vi "DSCProgClient.vi"() -> ()   [LabVIEW 2011]
uses:
  <vilib>/variable/tagger/epics/API/internal/List Records (By Ref).vi
  <vilib>/variable/tagger/epics/API/internal/Undeploy EPICS Client (By Ref).vi
  <vilib>/variable/tagger/epics/API/NI_EPICS_Client.lvlib
  <vilib>/lvdsc/NI_DSC.lvlib
panel:
  in  "network settings":T1={"use binding? (F)"=TRUE, "URL"="\\\\ndw1032\\vlinac\\css\\css:cos\\VAL", "access type"=enum."Read/write", "buffer size"=50, "use buffering? (F)"=FALSE, "single writer? (F)"=FALSE}
  out "error out 2":errorcluster
  out "data out":dbl
  out "error out":errorcluster={"status"=TRUE, "code"=-1967362038, "source"="Search Variable Container in DSCProgClient.vi"}
  out "records":string[](array[string])=["css:cos"]
  in  "stop":bool
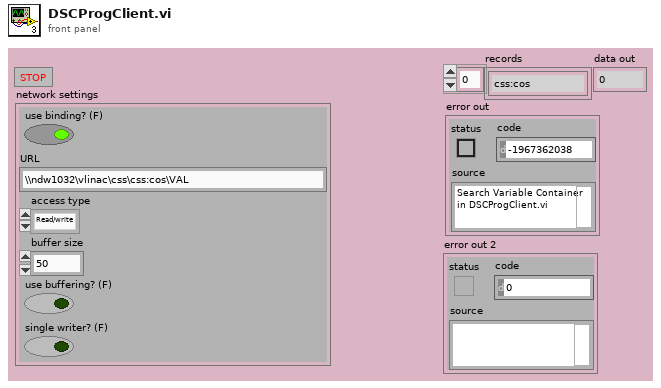
[diagram p1: front panel]
types:
  T1 = cluster{"use binding? (F)":bool, "URL":string, "access type":enum32{"Read only", "Write only", "Read/write"}, "buffer size":u32, "use buffering? (F)":bool, "single writer? (F)":bool}
  T2 = enum32{"u32BitField", "bool", "double", "string", "int8", "uint8", "int16", "uint16", "int32", "uint32", "int64", "uint64", "single", "double waveform", "int16 waveform", "array of boolean", "array of int8", "array of uint8", "array of int16", "array of uint16", "array of int32", "array of uint32", "array of int64", "array of uint64", "array of single", "array of double", "array of double waveform", "array of int16 waveform", "array of string", "variant", "timestamp", "fixed point", "custom"}
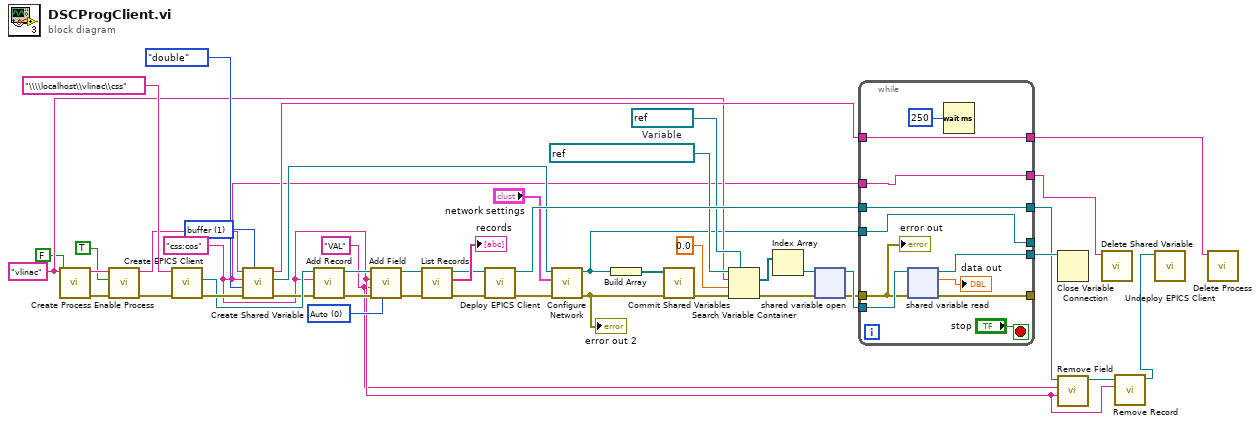
[diagram p0: block diagram]
diagram:
  w7 = u16 1 items=["commit", "buffer"] ("set mode")
  w34 = refnum<k21> refnum  # Variable
  w20 = "vlinac" ("process name")
  w45 = u16 0 items=["Auto", "Double", "Bool", "String", "Short", "Float", "Enum", "Long", "Array of Double"] ("data type")
  w1 = "VAL" ("field name")
  w2 = "css:cos" ("record name")
  n1 = call <vilib>:"Create Process.vi"("run?"=FALSE, "process name"=w20) -> ("error out"=w22:errorcluster, "process name out"=w26:string)  [unwired: 8 in]
  n2 = call <vilib>:"Enable Process.vi"("error in (no error)"=w22, "run?"=TRUE, "process name"=w26) -> ("error out"=w23:errorcluster, "process name out"=w25:string)  [unwired: 7 in]
  n3 = call <vilib>:"Create EPICS Client.vi"("error in (no error)"=w23, "EPICS Client URL in"="\\\\localhost\\vlinac\\css") -> ("error out"=w21:errorcluster, "EPICS Client ref"=w19:refnum<data-value>)  [unwired: 7 in, 1 out]
  n4 = call <vilib>:"Create Shared Variable.vi"("set mode"=w7, "error in (no error)"=w21, "data type"=T2."double", "shared variable name"=w2, "process name"=w25) -> ("error out"=w17:errorcluster, "shared variable"=w14:refnum<k21>, "process name out"=w37:string)  [unwired: 4 in]
  n5 = call <vilib>:"Add Record.vi"("error in (no error)"=w17, "record name"=w2, "EPICS Client ref in"=w19) -> ("error out"=w16:errorcluster, "EPICS Client ref out"=w18:refnum<data-value>)  [unwired: 5 in, 2 out]
  n6 = call <vilib>:"Add Field.vi"("data type"=w45, "error in (no error)"=w16, "field name"=w1, "record name"=w2, "EPICS Client ref in"=w18) -> ("error out"=w44:errorcluster, "EPICS Client ref out"=w43:refnum<data-value>)  [unwired: 3 in, 2 out]
  n7 = call-poly <vilib>:"List Records.vi"("error in (no error)"=w44, "EPICS Client ref in"=w43) -> ("error out"=w40:errorcluster, "records"=→"records":string[], "EPICS Client ref out"=w41:refnum<data-value>)  [unwired: 7 in]
  n8 = call <vilib>:"Deploy EPICS Client.vi"("error in (no error)"=w40, "EPICS Client ref in"=w41) -> ("error out"=w13:errorcluster, "EPICS Client ref out"=w39:refnum<data-value>)  [unwired: 8 in]
  n9 = call <vilib>:"Configure Network.vi"("error in (no error)"=w13, "network settings"="network settings", "variable reference in"=w14) -> ("error out"=w12:errorcluster, "variable reference out"=w9:refnum<k21>)  [unwired: 7 in]
  "error out 2" <- w12
  n10 = Build Array(w9) -> (w10:refnum<k21>[])
  n11 = call <vilib>:"Commit Shared Variables.vi"("error in (no error)"=w12, "shared variables"=w10) -> ("error out"=w11:errorcluster)  [unwired: 8 in, 1 out]
  n12 = Search Variable Container(7:w34, 8:w11, 9:0.0, 10:w20, 11:refnum<k21> "ni.var.psp://localhost/" ("container refnum in")) -> (0:w28:errorcluster, 2:w32:refnum<k21>[])  [unwired: 1 in, 1 out]
  n13 = Index Array(array=w32) -> (element=w29:refnum<k21>)  [unwired: 1 in]
  n14 = shared-variable-open(w29, w28) -> (w31:refnum<k21>, w27:errorcluster)  [unwired: 1 in]
  n15 = while {
    tunnel: w39 -> [w55]
    tunnel: [w55] -> w3
    tunnel: w37 -> [w54]
    tunnel: [w54] -> w36
    tunnel: w9 -> [w53]
    tunnel: [w53] -> _
    tunnel: w31 -> [w52]
    tunnel: [w50] -> w30
    tunnel: w27 -> [w48]
    tunnel: [w49] -> _
    tunnel: w2 -> [w47]
    tunnel: [w47] -> w8
    stop <- "stop" stop-if-true
    n16 = shared-variable-read(w52, w48) -> (w50:refnum<k21>, w49:errorcluster, →"data out":dbl)  [unwired: 1 out]
    n17 = Wait (ms)(milliseconds to wait=u32 250) -> ()  [unwired: 1 out]
    "error out" <- w48
  }
  n18 = Close Variable Connection(11:w30) -> ()  [unwired: 1 in, 1 out]
  n19 = call <vilib>:"Remove Field.vi"("record name"=w2, "field name"=w1, "EPICS Client ref in"=w3) -> ("EPICS Client ref out"=w5:refnum<data-value>)  [unwired: 7 in, 1 out]
  n20 = call <vilib>:"Delete Shared Variable.vi"("shared variable"=w8) -> ()  [unwired: 10 in, 1 out]
  n21 = call <vilib>:"Remove Record.vi"("record name"=w2, "EPICS Client ref in"=w5) -> ("EPICS Client ref out"=w4:refnum<data-value>)  [unwired: 8 in, 1 out]
  n22 = call-poly <vilib>:"Undeploy EPICS Client.vi"("EPICS Client ref"=w4) -> ()  [unwired: 10 in, 1 out]
  n23 = call <vilib>:"Delete Process.vi"("process name"=w36) -> ()  [unwired: 10 in, 1 out]
